vi "Time constant.vi"(10 "Numeric in":dbl, 11 "Cluster":T1) -> (3 "Numeric out":dbl)   [LabVIEW 2021]
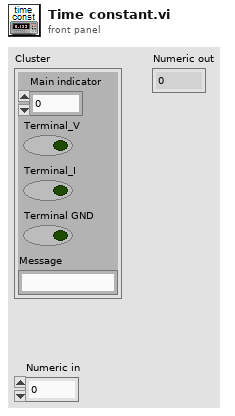
[diagram p1: front panel]
types:
  T1 = cluster{"Main indicator":dbl, "Terminal_V":bool, "Terminal_I":bool, "Terminal GND":bool, "Message":string}
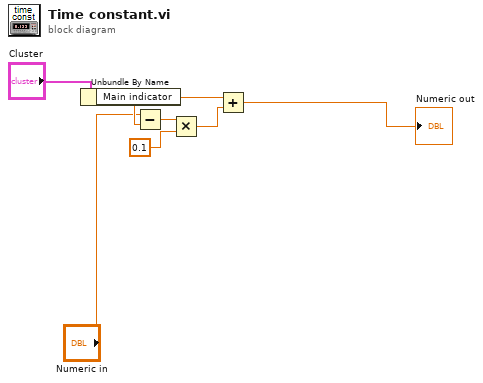
[diagram p0: block diagram]
diagram:
  n1 = Unbundle By Name("Cluster") -> ("Main indicator"=w6:dbl)
  n2 = Subtract(x="Numeric in", y=w6) -> (x-y=w1:dbl)
  n3 = Multiply(x=w1, y=0.1) -> (x*y=w3:dbl)
  n4 = Add(x=w6, y=w3) -> (x+y=→"Numeric out":dbl)
